vi "Radio Labeling and Difference Matrix Tester.vi"(2 "Difference Between Labels Matrix":i32[][](array[numeric]), 3 "Radio Labels":i32[](array[numeric])) -> (0 "Works?":bool, 1 "Working Labels Array":bool[][](array[boolean]))   [LabVIEW 2016]
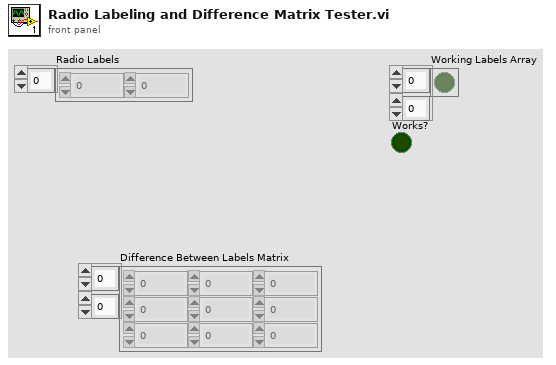
[diagram p1: front panel]
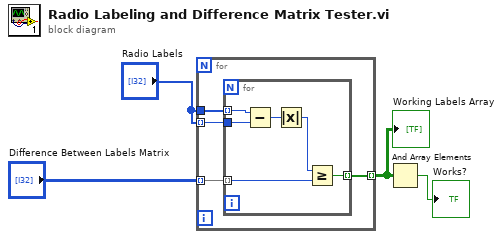
[diagram p0: block diagram]
diagram:
  n1 = for {
    tunnel: "Difference Between Labels Matrix" -> [w8] mode=indexing
    tunnel: "Radio Labels" -> [w7] mode=indexing
    tunnel: "Radio Labels" -> [w6]
    tunnel: [w5] -> w2 mode=indexing
    n2 = for {
      tunnel: w8 -> [w11] mode=indexing
      tunnel: w7 -> [w13]
      tunnel: w6 -> [w14] mode=indexing
      tunnel: [w9] -> w5 mode=indexing
      n3 = Subtract(x=w14, y=w13) -> (x-y=w12:i32)
      n4 = Absolute Value(x=w12) -> (abs(x)=w10:i32)
      n5 = Greater Or Equal?(x=w10, y=w11) -> (x >= y?=w9:bool)
    }
  }
  "Working Labels Array" <- w2
  n6 = And Array Elements(Boolean array=w2) -> (logical AND=→"Works?":bool)
